vi "Split (single).vi"(8 "error in (no error)":errorcluster, 9 "fractional index":dbl, 11 "XY-data":cluster{"X-array":dbl[], "Y-array":dbl[]} {"Y-array" format="%.2p"; "X-array" format="%.2p"}) -> (0 "error out":errorcluster, 2 "XY-data (B) out":cluster{"X-array":dbl[], "Y-array":dbl[]}, 3 "XY-data (A) out":cluster{"X-array":dbl[], "Y-array":dbl[]})   [LabVIEW 2019, in "xy_utilities.lvlib"]
doc: "Divides <B>XY-Data</B> at <b>index</b> (in units of the x array) and returns <B>XY-Data A</B> and <B>XY-Data B</B>.\n\nThe element at <b>index</b> will be at the beginning of <B>XY-Data B</B>\n\nWire data to the data input to determine the polymorphic instance to use or manually select the instance."
uses:
  xy_utilities.lvlib
  Sort (single).vi
  <userlib>/_OpenG.lib/array/array.llb/Sort Array__ogtk.vi
  <userlib>/_OpenG.lib/array/array.llb/Sort 1D Array (DBL)__ogtk.vi
  <userlib>/_OpenG.lib/array/array.llb/Reorder Array2__ogtk.vi
  <userlib>/_OpenG.lib/array/array.llb/Reorder 1D Array2 (DBL)__ogtk.vi
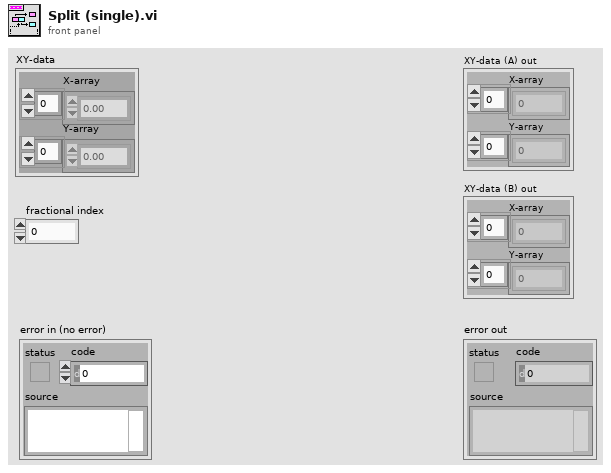
[diagram p1: front panel]
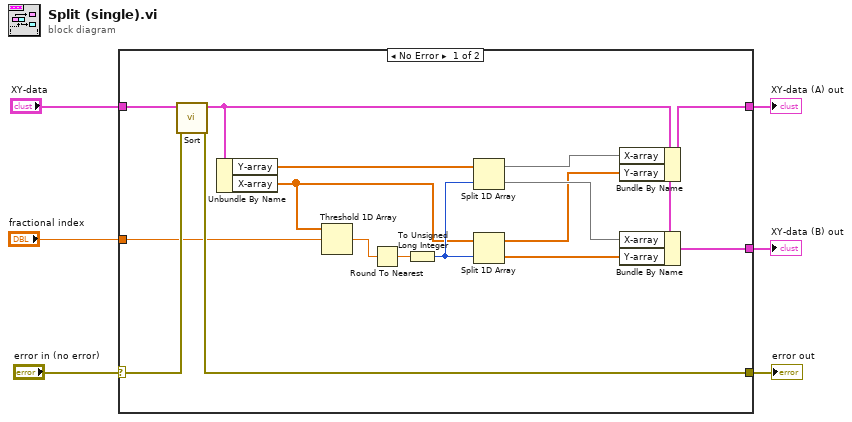
[diagram p0: block diagram]
diagram:
  n1 = case shown="No Error" "error in (no error)" {
    selector: "error in (no error)" -> [w14 w24]
    tunnel: [w13 w24] -> w5
    tunnel: "XY-data" -> [w15 w23]
    tunnel: [w17 w23] -> w3
    tunnel: [w18 _] -> w2
    tunnel: "fractional index" -> [w12 _]
    frame No Error {
      n2 = call-poly "Sort.vi"("error in (no error)"=w14, "XY-data"=w15) -> ("error out"=w13:errorcluster, "Sorted XY-data out"=w16:cluster{"X-array":dbl[], "Y-array":dbl[]})  [unwired: 7 in, 1 out]
      n3 = Unbundle By Name(w16) -> ("Y-array"=w8:dbl[], "X-array"=w7:dbl[])
      n4 = Threshold 1D Array(2:w12, 3:w7) -> (0:w11:dbl)  [unwired: 1 in]
      n5 = Round To Nearest(number=w11) -> (nearest integer value=w10:dbl)
      n6 = To Unsigned Long Integer(number=w10) -> (unsigned 32bit integer=w9:u32)
      n7 = Split 1D Array(array=w8, index=w9) -> (first subarray=w22:dbl[], second subarray=w21:dbl[])
      n8 = Split 1D Array(array=w7, index=w9) -> (first subarray=w20:dbl[], second subarray=w19:dbl[])
      n9 = Bundle By Name(cluster=w16, "X-array"=w22, "Y-array"=w20) -> (w17:cluster{"X-array":dbl[], "Y-array":dbl[]})
      n10 = Bundle By Name(cluster=w16, "X-array"=w21, "Y-array"=w19) -> (w18:cluster{"X-array":dbl[], "Y-array":dbl[]})
    }
    frame Error {
    }
  }
  "error out" <- w5
  "XY-data (A) out" <- w3
  "XY-data (B) out" <- w2
